vi "BGA244_init.vi"(8 "error in":errorcluster, 11 "VISA in":refnum<visa-resource-name>="COM24") -> (0 "error out":errorcluster, 1 "status":bool, 3 "VISA out":refnum<visa-resource-name>)   [LabVIEW 2019]
uses:
  <vilib>/Instr/_visa.llb/VISA Configure Serial Port (Instr).vi
panel:
  out "sn_build":string
  out "IDN":string
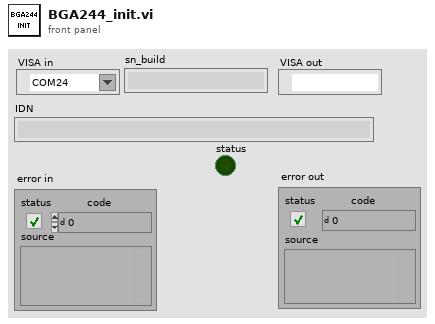
[diagram p1: front panel]
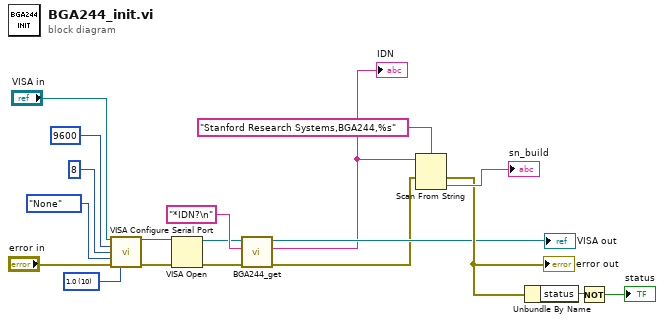
[diagram p0: block diagram]
diagram:
  w16 = u16 10 items=["1.0"=10, "1.5"=15, "2.0"=20] ("stop bits (10: 1 bit)")
  n1 = call-poly "VISA Configure Serial Port"("VISA resource name"="VISA in", "baud rate (9600)"=u32 9600, "data bits (8)"=u16 8, "parity (0:none)"=enum16{"None", "Odd", "Even", "Mark", "Space"}."None", "error in (no error)"="error in", "stop bits (10: 1 bit)"=w16) -> ("VISA resource name out"=w13:refnum<visa-resource-name>, "error out"=w12:errorcluster)  [unwired: 8 in]
  n2 = VISA Open(error in (no error)=w12, VISA resource name=w13) -> (VISA resource name=w3:refnum<visa-resource-name>, error out=w2:errorcluster)  [unwired: 3 in]
  n3 = call "BGA244_get.vi"("error in"=w2, "string in"="*IDN?\n", "VISA in"=w3) -> ("error out"=w5:errorcluster, "string out"=w1:string, "VISA out"=→"VISA out":refnum<visa-resource-name>)  [unwired: 6 in]
  "IDN" <- w1
  n4 = Scan From String(format string="Stanford Research Systems,BGA244,%s", input string=w1, error in=w5) -> (error out=w9:errorcluster, output 1=→"sn_build":string)  [unwired: 2 in, 2 out]
  "error out" <- w9
  n5 = Unbundle By Name(w9) -> ("status"=w8:bool)
  n6 = Not(x=w8) -> (.not. x?=→"status":bool)
